vi "test_Format Instrument String Command_Format array command(comma delimited, default).vi"(8 "error in (no error)":errorcluster, 11 "TestCase in":refnum<class "Instrument Addon Unit Tests.lvclass">) -> (0 "error out":errorcluster, 3 "TestCase out":refnum<class "Instrument Addon Unit Tests.lvclass">)   [LabVIEW 2018, in "Instrument Addon Unit Tests.lvclass"]
uses:
  Instrument Addon Unit Tests.lvclass
  <vilib>/addons/_JKI Toolkits/VI Tester/TestCase.llb/TestCase.lvclass
  Addon/Addon Engine/Instrument Addon Engine.lvlib
  Addon/Addon Shared/Types/Linked Channel Cluster.ctl
  Addon/Addon Shared/Instrument Addon Shared.lvlib
  Addon/Addon Shared/Types/Command Parameters.ctl
  Addon/Addon Shared/Types/Endian.ctl
  Addon/Addon Shared/Types/Type Cast Type.ctl
  Addon/Addon Shared/Types/Metadata Channel Type.ctl
  Addon/Addon Shared/Types/Protocol Data Type.ctl
  Addon/Addon Shared/Types/MetaData Parameters.ctl
  Addon/Addon Shared/Types/Meta Data RT Configuration Cluster.ctl
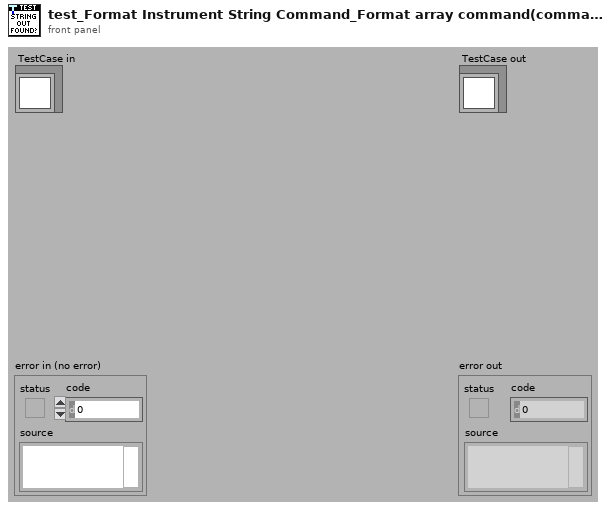
[diagram p1: front panel]
types:
  T1 = typedef "Instrument Addon Shared.lvlib/Meta Data RT Configuration Cluster.ctl" = cluster{"MetaData Parameters":T2, "Data Index":i32, "Data Length":i32}
  T2 = typedef "Instrument Addon Shared.lvlib/MetaData Parameters.ctl" = cluster{"Data Type":T3, "Channel Type":T4, "List":string[], "Format String":string, "Type":T5, "Delimiter":string, "Endian":T6}
  T3 = typedef "Instrument Addon Shared.lvlib/Protocol Data Type.ctl" = enum16{"Single Channel", "Array"}
  T4 = typedef "Instrument Addon Shared.lvlib/Metadata Channel Type.ctl" = enum16{"Enumerated List", "Format", "Type Cast"}
  T5 = typedef "Instrument Addon Shared.lvlib/Type Cast Type.ctl" = enum16{"DBL", "SGL", "U64", "U32", "U16", "U8", "I64", "I32", "I16", "I8"}
  T6 = typedef "Instrument Addon Shared.lvlib/Endian.ctl" = enum16{"Native", "Little", "Big"}
  T7 = typedef "Instrument Addon Shared.lvlib/Command Parameters.ctl" = cluster{"Command":string, "Linked Channels":T8[], "Pad":bool, "Length":u32, "Pad Value":u8}
  T8 = typedef "Instrument Addon Shared.lvlib/Linked Channel Cluster.ctl" = cluster{"Variable Name":string, "GUID":string}
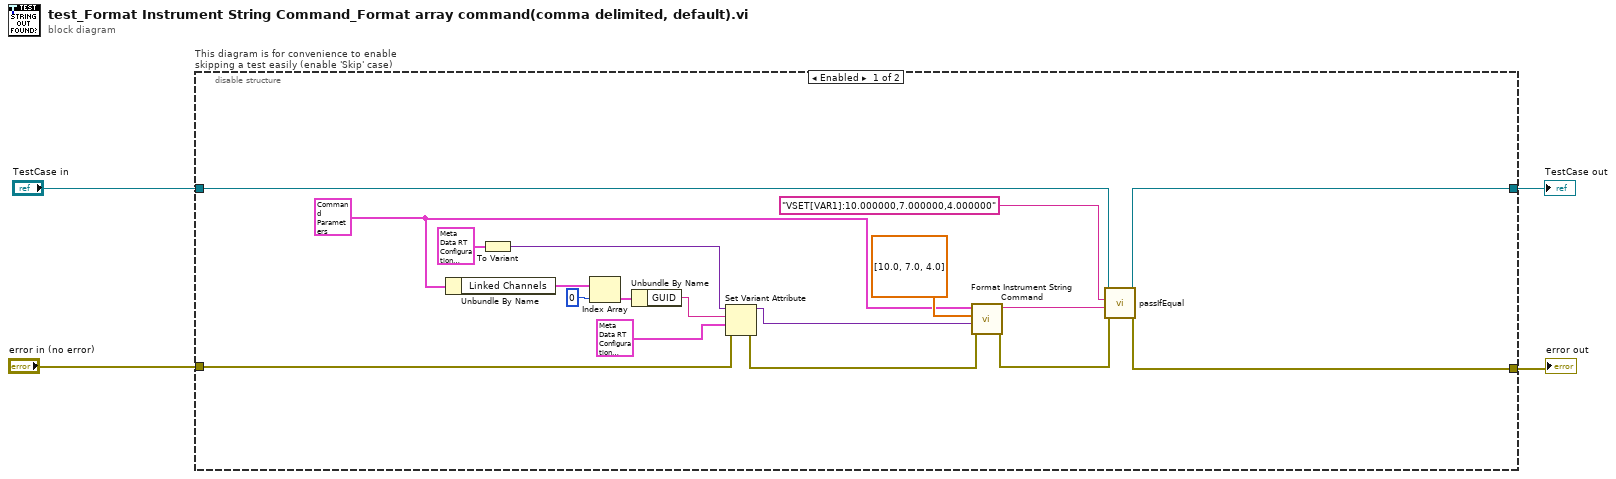
[diagram p0: block diagram]
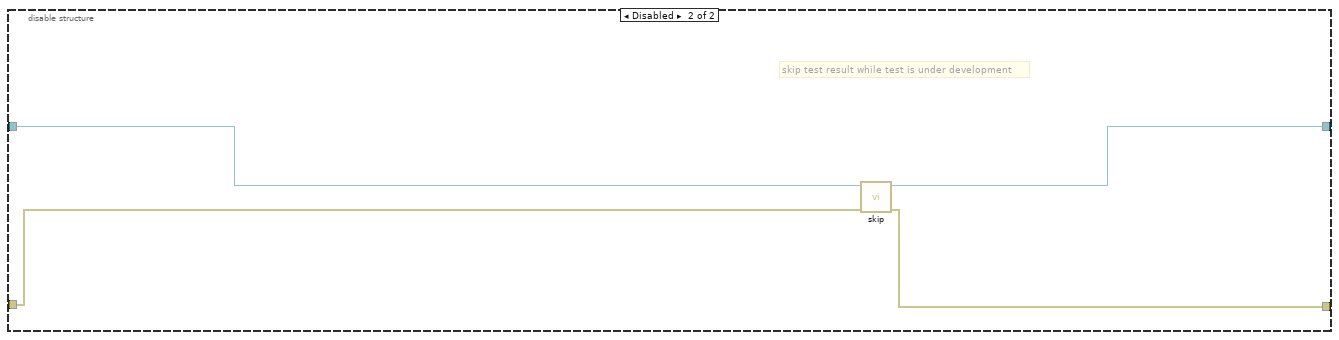
[diagram p2: hidden frame]
diagram:
  n1 = disable-structure "This diagram is for convenience to enable skipping a test easily (enable 'Skip' case)" shown="Enabled" {
    disable-tunnel: "TestCase in" -> [w22 w26]
    disable-tunnel: [w5 w24] -> w1
    disable-tunnel: [w21 w25] -> w3
    disable-tunnel: "error in (no error)" -> [w7 w23]
    frame Enabled {
      w13 = T7 {"Command"="VSET[VAR1]:[MetadataChannel]", "Linked Channels"=[{"Variable Name"="MetadataChannel", "GUID"="9428600d-6a85-43b8-aaac-a755da7e0c9b"}], "Pad"=FALSE, "Length"=0, "Pad Value"=0} ("Command Parameters")
      n2 = Unbundle By Name(w13) -> ("Linked Channels"=w12:T8[])
      n3 = To Variant(anything=T1 {"MetaData Parameters"={"Data Type"=enum."Single Channel", "Channel Type"=enum."Enumerated List", "List"=[], "Format String"="", "Type"=enum."DBL", "Delimiter"="", "Endian"=enum."Native"}, "Data Index"=0, "Data Length"=0}) -> (Variant=w18:variant)
      n4 = Index Array(array=w12, index=0) -> (element=w10:T8)
      n5 = Unbundle By Name(w10) -> ("GUID"=w9:string)
      n6 = Set Variant Attribute(Variant=w18, name=w9, value=T1 {"MetaData Parameters"={"Data Type"=enum."Array", "Channel Type"=enum."Format", "List"=[], "Format String"="", "Type"=enum."DBL", "Delimiter"=",", "Endian"=enum."Native"}, "Data Index"=0, "Data Length"=3}, error in=w7) -> (Variant out=w17:variant, error out=w6:errorcluster)  [unwired: 1 out]
      n7 = call "Format Instrument String Command.vi"("error in (no error)"=w6, "MetaData Lookup in"=w17, "MetaData"=dbl[] [10.0, 7.0, 4.0], "Command Parameters"=w13) -> ("error out"=w20:errorcluster, "Command"=w15:string)  [unwired: 5 in, 1 out]
      n8 = call-dynamic "passIfEqual.vi"("error in (no error)"=w20, "y"=w15, "x"="VSET[VAR1]:10.000000,7.000000,4.000000" ("Command"), "TestCase in"=w22) -> ("error out"=w21:errorcluster, "TestCase out"=w5:refnum<class "Instrument Addon Unit Tests.lvclass">)  [unwired: 6 in]
    }
    frame Disabled {
      # "skip test result while test is under development"
      n9 = call <vilib>:"skip.vi"("error in (no error)"=w23, "TestCase in"=w26) -> ("error out"=w25:errorcluster, "TestCase out"=w24:refnum<class "Instrument Addon Unit Tests.lvclass">)  [unwired: 8 in]
    }
  }
  "error out" <- w3
  "TestCase out" <- w1
